vi "Dispose Stop.vi"(8 "error in (no error)":errorcluster, 11 "Thread in":refnum<class "Thread.lvclass">) -> (0 "error out":errorcluster, 3 "Thread out":refnum<class "Thread.lvclass">)   [LabVIEW 2021, in "DSF Core.lvlib" / "Thread.lvclass"]
uses:
  Thread.lvclass
  Thread.lvclass/Thread.ctl
  <vilib>/NI/Memory Manager/Classes/Pointer/Pointer.lvclass/Pointer.ctl
  <vilib>/NI/Memory Manager/Classes/Pointer/Get Internal.vi
  <vilib>/NI/Memory Manager/Classes/Pointer/Errors.vi
  <vilib>/NI/Memory Manager/Classes/Pointer/Zone.vi
  <vilib>/NI/Memory Manager/Classes/Pointer/Set Address.vi
  <vilib>/NI/Memory Manager/Classes/Pointer/Set Size.vi
  <vilib>/NI/Memory Manager/Classes/Pointer/Set Internal.vi
  <vilib>/NI/Memory Manager/Classes/Pointer/Get Address.vi
  <vilib>/NI/Memory Manager/Classes/Pointer/Check Null Pointer.vi
  <vilib>/NI/Memory Manager/Classes/Pointer/Create Error.vi
  <vilib>/NI/Memory Manager/Classes/Pointer/Null Pointer.vi
  <vilib>/NI/Memory Manager/Classes/Pointer/Is Null.vi
  <vilib>/NI/Memory Manager/VIs/New Error Cluster.vi
  <vilib>/NI/Memory Manager/VIs/New Error Cluster (512B).vi
  <vilib>/NI/Memory Manager/VIs/Set Error Status.vi
  <vilib>/NI/Memory Manager/VIs/Set Error Code.vi
  <vilib>/NI/Memory Manager/VIs/Set Error Source.vi
  <vilib>/NI/Memory Manager/Constants/Constants.vi
  <vilib>/NI/Memory Manager/Constants/Library Name.vi
  <vilib>/NI/Memory Manager/Classes/Pointer/Pointer Error Info.vi
  <vilib>/NI/Memory Manager/VIs/Write String to Source.vi
  <vilib>/NI/Memory Manager/Constants/Pointer Class Name.vi
  <vilib>/NI/Memory Manager/Classes/Pointer/Pointer.lvclass
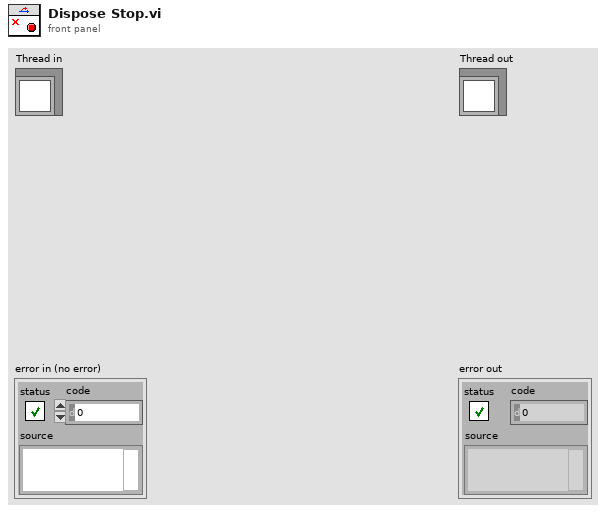
[diagram p1: front panel]
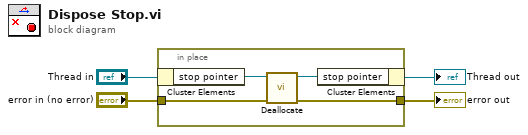
[diagram p0: block diagram]
diagram:
  n1 = in-place {
    in-place-border: "error in (no error)" -> [w8]
    in-place-border: [w7] -> w3
    n2 = in-place-cluster #1("Thread in") -> ("stop pointer"=w6:refnum<class "Pointer.lvclass">)
    n3 = call <vilib>:"Deallocate.vi"("error in (no error)"=w8, "Pointer"=w6) -> ("error out"=w7:errorcluster, "Pointer type"=w5:refnum<class "Pointer.lvclass">)  [unwired: 8 in]
    n4 = in-place-cluster #1("stop pointer"=w5) -> (→"Thread out":refnum<class "Thread.lvclass">)
  }
  "error out" <- w3
